vi "FindIslandBounds.vi"(6 "IslandSize":dbl, 8 "yMax":dbl, 9 "yMin":dbl, 10 "xMax":dbl, 11 "xMin":dbl) -> (3 "Bounds":cluster{dbl[][]}[](array[cluster]))   [LabVIEW 2014]
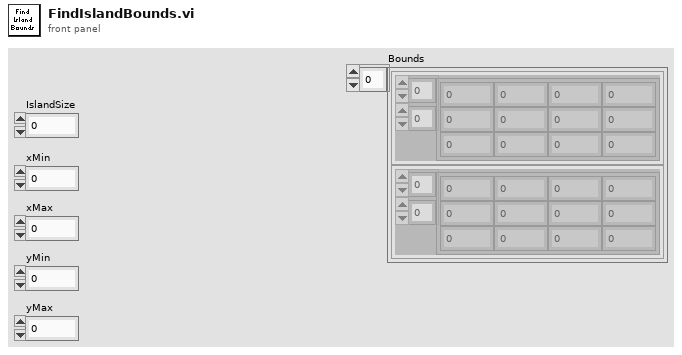
[diagram p1: front panel]
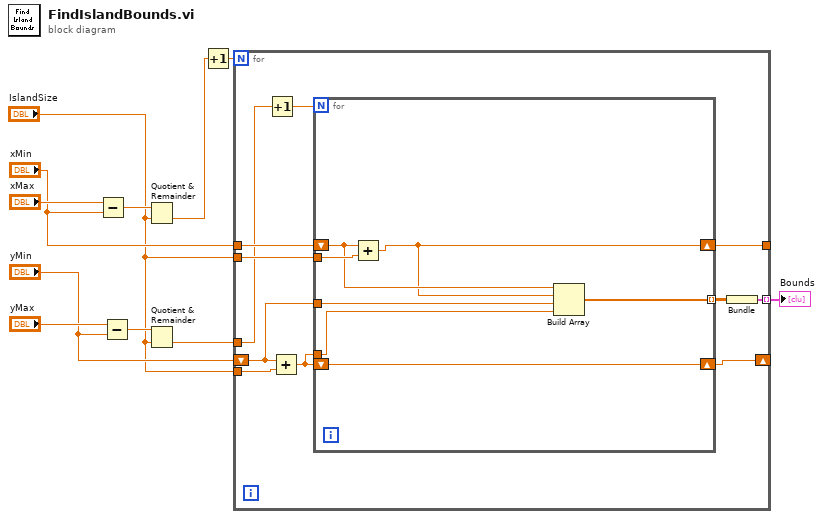
[diagram p0: block diagram]
diagram:
  n1 = Subtract(x="xMax", y="xMin") -> (x-y=w10:dbl)
  n2 = Subtract(x="yMax", y="yMin") -> (x-y=w8:dbl)
  n3 = Quotient & Remainder(x=w10, y="IslandSize") -> (floor(x/y)=w2:dbl)  [unwired: 1 out]
  n4 = Quotient & Remainder(x=w8, y="IslandSize") -> (floor(x/y)=w7:dbl)  [unwired: 1 out]
  n5 = Increment(x=w2) -> (x+1=w1:dbl)
  n6 = for {
    N: w1 -> [_]
    tunnel: w7 -> [w12]
    tunnel: "IslandSize" -> [w21]
    shift-right: [w18] -> _
    shift-left: "yMin" -> [w17]
    tunnel: "IslandSize" -> [w19]
    tunnel: [w14] -> w3 mode=indexing
    tunnel: "xMin" -> [w22]
    tunnel: [w20] -> _
    n7 = Increment(x=w12) -> (x+1=w13:dbl)
    n8 = Add(x=w17, y=w19) -> (x+y=w16:dbl)
    n9 = for {
      N: w13 -> [_]
      shift-right: [w26] -> w20
      shift-left: w22 -> [w27]
      tunnel: w21 -> [w29]
      shift-right: [w28] -> w18
      shift-left: w16 -> [w28]
      tunnel: w17 -> [w25]
      tunnel: w16 -> [w24]
      tunnel: [w23] -> w15 mode=indexing
      n10 = Add(x=w27, y=w29) -> (x+y=w26:dbl)
      n11 = Build Array(w27, w26, w25, w24) -> (w23:dbl[])
    }
    n12 = Bundle(w15) -> (w14:cluster{dbl[][]})  [unwired: 1 in]
  }
  "Bounds" <- w3
